vi "Read Config.vi"(8 "error in (no error)":errorcluster, 11 "SOL-Server in":refnum<class "SOL-Server.lvclass">) -> (0 "error out":errorcluster, 3 "SOL-Server out":refnum<class "SOL-Server.lvclass">)   [LabVIEW 2020, in "Summer of LabVIEW.lvlib" / "SOL-Server.lvclass"]
uses:
  SOL-Server.lvclass
  SOL-Server.lvclass/SOL-Server.ctl
  SOL-Config/SOL-Config.lvclass
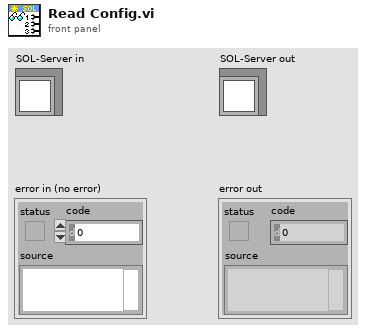
[diagram p1: front panel]
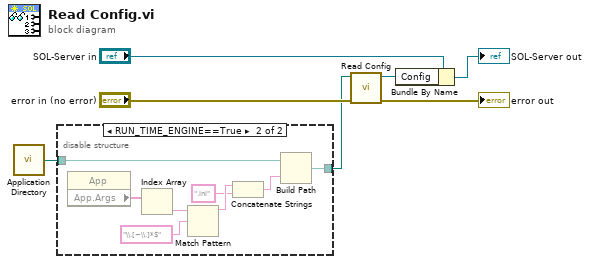
[diagram p0: block diagram]
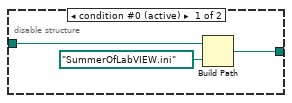
[diagram p2: hidden frame]
diagram:
  n1 = call <vilib>:"Application Directory.vi"() -> ("Application Directory"=w6:path)
  n2 = disable-structure shown="RUN_TIME_ENGINE==True" {
    disable-tunnel: w6 -> [w10 w13]
    disable-tunnel: [w8 w11] -> w3
    frame condition #0 (active) {
      n3 = Build Path(base path=w10, name or relative path=path "SummerOfLabVIEW.ini") -> (appended path=w8:path)
    }
    frame condition #1 {
      n4 = property class="App"() -> ("App.Args"=w18:string[])  [unwired: 2 in, 2 out]
      n5 = Index Array(array=w18) -> (element=w17:string)  [unwired: 1 in]
      n6 = Match Pattern(string=w17, regular expression="\\.[~\\.]*$") -> (before substring=w15:string)  [unwired: 4 out]
      n7 = Concatenate Strings(w15, ".ini" ("string")) -> (w12:string)
      n8 = Build Path(base path=w13, name or relative path=w12) -> (appended path=w11:path)
    }
  }
  n9 = call "Read Config.vi"("error in (no error)"="error in (no error)", "INI"=w3) -> ("error out"=→"error out":errorcluster, "SOL-Config out"=w1:refnum<class "SOL-Config.lvclass">)  [unwired: 8 in]
  n10 = Bundle By Name(cluster="SOL-Server in", "Config"=w1) -> (→"SOL-Server out":refnum<class "SOL-Server.lvclass">)
